vi "Host_PC.vi"() -> ()   [LabVIEW 2011]
uses:
  <vilib>/NXT/NXT Controls/ConnectionType.ctl
panel:
  in  "number":i32
  out "resulting string":string
  in  "input 1":i32
  out "NXT Seconds Elapsed":string="0"
  in  "Connection type":T1
  in  "NXT name":string="MyNXT"
  out "Is Paired?":bool
  in  "stop":bool
  # "Steps:\n1. Connect NXT Motor NXT Port A\n2. Download and run Client_NXT.vi on the NXT.\n3. Set NXT Name and Connection Type appropriately on this VI.\n4. Run this VI.\n5. Use the Speed dial to adjust the motor speed on the NXT."
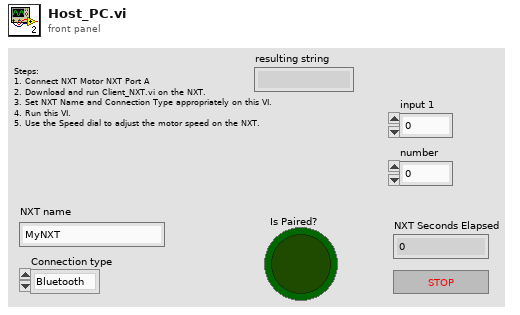
[diagram p1: front panel]
types:
  T1 = typedef "ConnectionType.ctl" = enum16{"Bluetooth", "USB", "WiFi"}
  T2 = typedef "nxt.ctl" = cluster{"nxtHandle":u32, "fileHandle":u32, "fileIterHandle":u32, "moduleHandle":u32, "modIterHandle":u32, "nxtIterHandle":u32}
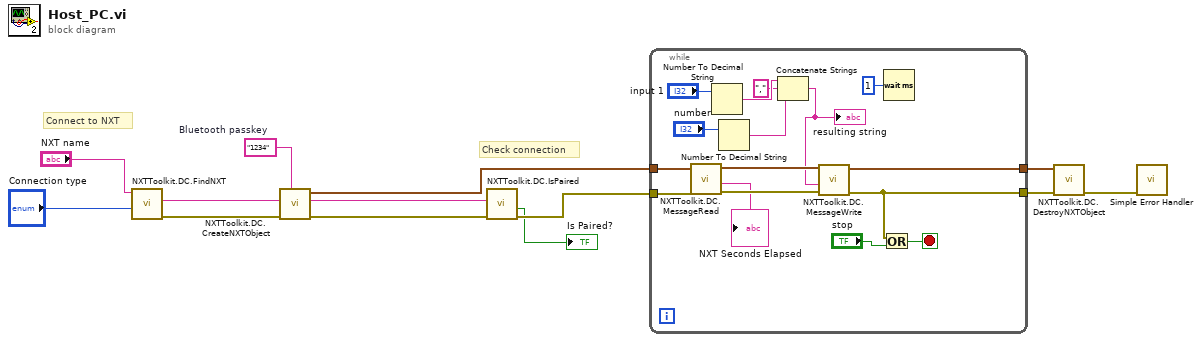
[diagram p0: block diagram]
diagram:
  w10 = "1234"  # Bluetooth passkey
  # "Check connection"
  # "Connect to NXT"
  n1 = call <vilib>:"NXTToolkit.DC.FindNXT.vi"("Connection type (USB)"="Connection type", "NXT name"="NXT name") -> ("error out"=w9:errorcluster, "VISA resource string"=w8:string)  [unwired: 7 in, 1 out]
  n2 = call <vilib>:"NXTToolkit.DC.CreateNXTObject.vi"("Bluetooth passkey (1234)"=w10, "error in (no error)"=w9, "VISA resource string (\"\" : find USB brick)"=w8) -> ("error out"=w7:errorcluster, "VISA resource string out"=w6:string, "NXTObject"=w4:T2)  [unwired: 6 in]
  n3 = call <vilib>:"NXTToolkit.DC.IsPaired.vi"("error in (no error)"=w7, "VISA resource string"=w6) -> ("error out"=w3:errorcluster, "Is Paired?"=→"Is Paired?":bool)  [unwired: 7 in, 1 out]
  n4 = while {
    tunnel: w3 -> [w22]
    tunnel: [w25] -> w12
    tunnel: w4 -> [w24]
    tunnel: [w26] -> w11
    stop <- w27 stop-if-true
    n5 = call <vilib>:"NXTToolkit.DC.MessageRead.vi"("error in (no error)"=w22, "NXTObject"=w24) -> ("error out"=w21:errorcluster, "Message"=→"NXT Seconds Elapsed":string, "NXTObject dup"=w23:T2)  [unwired: 4 in, 3 out]
    n6 = Number To Decimal String(number="input 1") -> (decimal integer string=w18:string)  [unwired: 1 in]
    n7 = Number To Decimal String(number="number") -> (decimal integer string=w17:string)  [unwired: 1 in]
    n8 = Concatenate Strings(w18, "," ("string"), w17) -> (w15:string)
    "resulting string" <- w15
    n9 = call <vilib>:"NXTToolkit.DC.MessageWrite.vi"("error in (no error)"=w21, "Message"=w15, "NXTObject"=w23) -> ("error out"=w25:errorcluster, "NXTObject dup"=w26:T2)  [unwired: 5 in, 2 out]
    n10 = Or(x=w25, y="stop") -> (x .or. y?=w27:bool)
    n11 = Wait (ms)(milliseconds to wait=u32 1) -> ()  [unwired: 1 out]
  }
  n12 = call <vilib>:"NXTToolkit.DC.DestroyNXTObject.vi"("error in (no error)"=w12, "NXTObject"=w11) -> ("error out"=w13:errorcluster)  [unwired: 9 in]
  n13 = call <vilib>:"Simple Error Handler.vi"("error in (no error)"=w13) -> ()  [unwired: 4 in, 5 out]
